vi "Get Oldest File in Directory.vi"(8 "error in":errorcluster, 11 "Directory":path) -> (0 "error out":errorcluster, 3 "Oldest File":path)   [LabVIEW 2018, in "Embedded Data Logger System Tests.lvclass"]
uses:
  Embedded Data Logger System Tests.lvclass
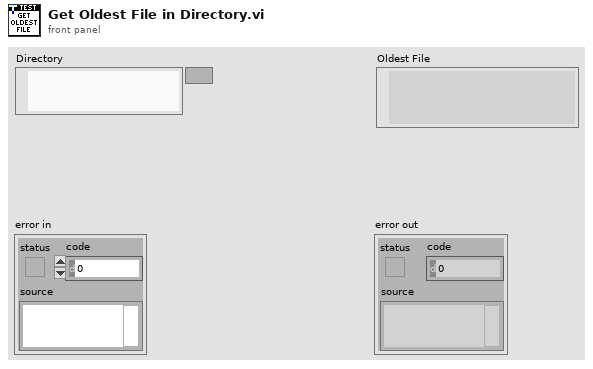
[diagram p1: front panel]
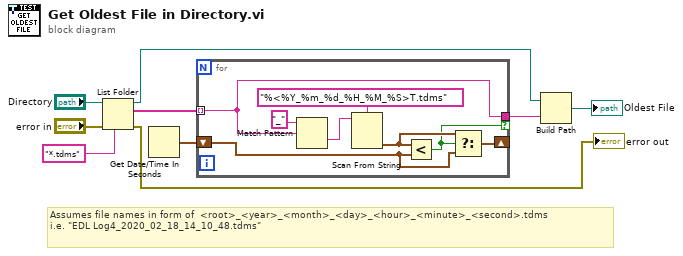
[diagram p0: block diagram]
diagram:
  # "Assumes file names in form of  <root>_<year>_<month>_<day>_<hour>_<minute>_<second>.tdms\ni.e. \"EDL Log4_2020_02_18_14_10_48.tdms\""
  n1 = List Folder(path="Directory", pattern="*.tdms", error in="error in") -> (path out=w6:path, filenames=w3:string[], error out=→"error out":errorcluster)  [unwired: 1 in, 1 out]
  n2 = Get Date/Time In Seconds() -> (seconds since 1Jan1904=w4:timestamp)
  n3 = for {
    tunnel: w3 -> [w10] mode=indexing
    shift-right: [w14] -> _
    shift-left: w4 -> [w15]
    tunnel: [w10] -> w5 if=w13
    n4 = Match Pattern(string="_", regular expression=w10) -> (after substring=w12:string)  [unwired: 1 in, 3 out]
    n5 = Scan From String(format string="%<%Y_%m_%d_%H_%M_%S>T.tdms", input string=w12) -> (output 1=w16:timestamp)  [unwired: 3 in, 3 out]
    n6 = Less?(x=w16, y=w15) -> (x < y?=w13:bool)
    n7 = Select(t=w16, s=w13, f=w15) -> (s? t:f=w14:timestamp)
  }
  n8 = Build Path(base path=w6, name or relative path=w5) -> (appended path=→"Oldest File":path)
